vi "SDR.vi"(0 "instrument handle":refnum<k15>="PXI1Slot2 (33)", 1 "Rm (ohm)":dbl=26118.0, 2 "MLC SLV (V)":dbl=2.0, 3 "Step Size":cluster{"WLV":dbl, "BLV":dbl, "SLV":dbl}={"WLV"=0.06, "BLV"=0.4, "SLV"=0.15000000000000002} {"SLV" format="%#_13g"; "BLV" format="%#_13g"; "WLV" format="%#_13g"}, 4 "RM (ohm)":dbl=39476.0, 5 "error in (no error)":errorcluster, 6 "Max fine attempts":i32=20, 8 "RMM (ohm)":dbl=10000000000.0, 9 "Rmm (ohm)":dbl=15300.0, 10 "MLC BLV (V)":dbl=2.0, 11 "MLC WLV (V)":dbl=2.26) -> (7 "BL voltage (V)":dbl=2.8, 12 "SL voltage (V)":dbl=2.15, 13 "WL voltage (V)":dbl=2.26, 14 "instrument handle out":refnum<k15>="PXI1Slot2 (33)", 15 "final resistance (ohm)":dbl=31406.349555562472 format="%#_6p", 17 "target hit?":bool=TRUE, 18 "final current (A)":dbl=6.368139017435645e-06, 19 "error out":errorcluster)   [LabVIEW 2018]
uses:
  Globals.vi
panel:
  out "attempt number":i32=1
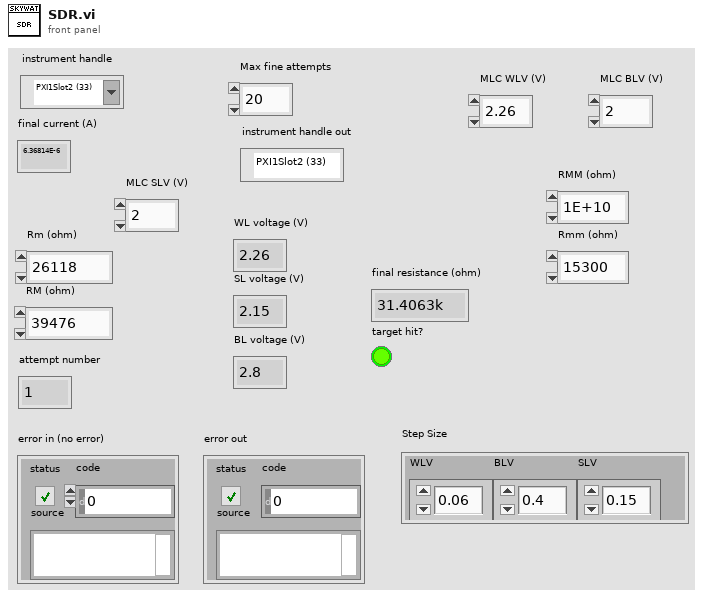
[diagram p1: front panel]
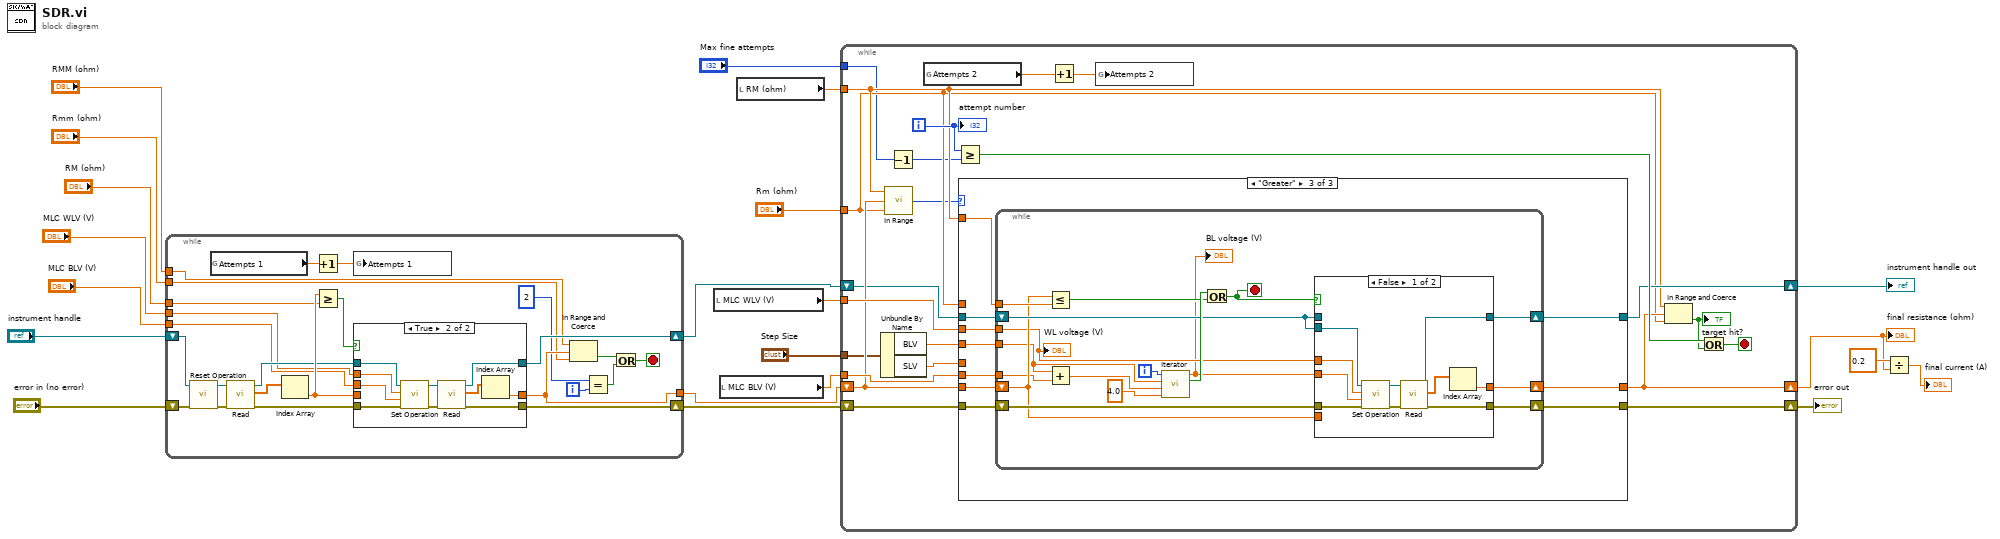
[diagram p0: block diagram]
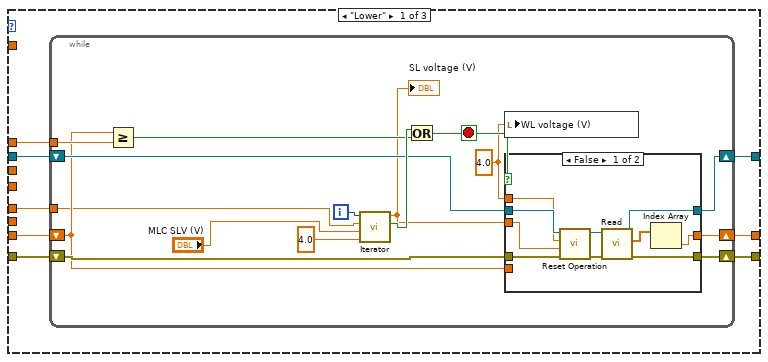
[diagram p3: hidden frame]
diagram:
  n1 = while {
    tunnel: [w36] -> w13
    tunnel: "RM (ohm)" -> [w33]
    shift-right: [w34] -> w11
    shift-left: "error in (no error)" -> [w38]
    shift-right: [w35] -> w12
    shift-left: "instrument handle" -> [w37]
    tunnel: "MLC WLV (V)" -> [w28]
    tunnel: "MLC BLV (V)" -> [w27]
    tunnel: "RMM (ohm)" -> [w26]
    tunnel: "Rmm (ohm)" -> [w25]
    i -> [w30]
    stop <- w32 stop-if-true
    n2 = call "Reset Operation.vi"("error in (no error)"=w38, "instrument handle"=w37) -> ("error out"=w41:errorcluster, "instrument handle out"=w39:refnum<k15>)  [unwired: 8 in]
    n3 = global read "Globals.vi" "Attempts 1"() -> (w23:dbl)
    n4 = call "Read.vi"("error in (no error)"=w41, "instrument handle"=w39) -> ("error out"=w42:errorcluster, "resistances (ohm)"=w40:dbl[], "instrument handle out"=w43:refnum<k15>)  [unwired: 6 in, 1 out]
    n5 = Index Array(array=w40) -> (element=w44:dbl)  [unwired: 1 in]
    n6 = Increment(x=w23) -> (x+1=w22:dbl)
    n7 = Greater Or Equal?(x=w44, y=w33) -> (x >= y?=w45:bool)
    n8 = global write "Globals.vi" "Attempts 1"(w22) -> ()
    n9 = case shown="True" w45 {
      tunnel: w42 -> [w48 w52]
      tunnel: [w48 w54] -> w34
      tunnel: w44 -> [w47 _]
      tunnel: [w47 w55] -> w36
      tunnel: w43 -> [w46 w58]
      tunnel: [w46 w56] -> w35
      tunnel: w28 -> [_ w50]
      tunnel: w27 -> [_ w49]
      frame False {
      }
      frame True {
        n10 = call "Set Operation.vi"("error in (no error)"=w52, "BLV"=w49, "WLV"=w50, "instrument handle"=w58) -> ("error out"=w53:errorcluster, "instrument handle out"=w57:refnum<k15>)  [unwired: 6 in]
        n11 = call "Read.vi"("error in (no error)"=w53, "instrument handle"=w57) -> ("error out"=w54:errorcluster, "resistances (ohm)"=w51:dbl[], "instrument handle out"=w56:refnum<k15>)  [unwired: 6 in, 1 out]
        n12 = Index Array(array=w51) -> (element=w55:dbl)  [unwired: 1 in]
      }
    }
    n13 = In Range and Coerce(upper limit=w26, x=w36, lower limit=w25) -> (In Range?=w24:bool)  [unwired: 1 out]
    n14 = Equal?(x=2, y=w30) -> (x = y?=w31:bool)
    n15 = Or(x=w24, y=w31) -> (x .or. y?=w32:bool)
  }
  n16 = local read "MLC WLV (V)"() -> (w7:dbl)
  n17 = local read "MLC BLV (V)"() -> (w6:dbl)
  n18 = local read "RM (ohm)"() -> (w9:dbl)
  n19 = while {
    shift-right: [w75] -> w16
    shift-left: w12 -> [w69]
    shift-right: [w74] -> w21
    shift-left: w11 -> [w68]
    tunnel: "Max fine attempts" -> [w60]
    tunnel: w9 -> [w71]
    tunnel: w7 -> [w73]
    tunnel: w6 -> [w72]
    tunnel: "Rm (ohm)" -> [w67]
    tunnel: "Step Size" -> [w63]
    shift-right: [w76] -> w18
    shift-left: w13 -> [w70]
    i -> [w79]
    stop <- w80 stop-if-true
    n20 = Unbundle By Name(w63) -> ("BLV"=w65:dbl, "SLV"=w64:dbl)
    n21 = call "In Range.vi"("Lower resistance (ohm)"=w67, "Resistance (ohm)"=w70, "Upper resistance (ohm)"=w71) -> ("range"=w66:enum16{"Lower", "In Range", "Greater"})
    n22 = Decrement(x=w60) -> (x-1=w59:i32)
    n23 = global read "Globals.vi" "Attempts 2"() -> (w61:dbl)
    n24 = Greater Or Equal?(x=w79, y=w59) -> (x >= y?=w78:bool)
    n25 = case shown="\"Greater\"" w66 {
      tunnel: w65 -> [_ _ w130]
      tunnel: w68 -> [w82 w119 w129]
      tunnel: [w86 w119 w128] -> w74
      tunnel: [w87 w120 w127] -> w75
      tunnel: [w81 w118 w123] -> w76
      tunnel: w71 -> [_ _ w126]
      tunnel: w69 -> [w84 w120 w125]
      tunnel: w70 -> [w85 w118 w124]
      tunnel: w67 -> [w88 _ _]
      tunnel: w73 -> [_ _ w122]
      tunnel: w72 -> [_ _ w121]
      tunnel: w64 -> [w83 _ _]
      frame "Lower" {
        n26 = while {
          shift-right: [w99] -> w87
          shift-left: w84 -> [w97]
          shift-right: [w100] -> w86
          shift-left: w82 -> [w98]
          tunnel: w88 -> [w93]
          shift-right: [w91] -> w81
          shift-left: w85 -> [w92]
          tunnel: w83 -> [w90]
          i -> [w104]
          stop <- w96 stop-if-true
          w94 = 4.0 ("level (V)")
          n27 = Greater Or Equal?(x=w92, y=w93) -> (x >= y?=w101:bool)
          n28 = call "Iterator.vi"("Final Value"=4.0 ("y"), "Initial Value"="MLC SLV (V)", "Step"=w90, "i"=w104) -> ("End Loop"=w102:bool, "Current Value"=w95:dbl)  [unwired: 6 in]
          "SL voltage (V)" <- w95
          n29 = Or(x=w102, y=w101) -> (x .or. y?=w96:bool)
          n30 = local write "WL voltage (V)"(w94) -> ()
          n31 = case shown="False" w96 {
            tunnel: w95 -> [w105 _]
            tunnel: [w112 w117] -> w100
            tunnel: [w111 w115] -> w99
            tunnel: w94 -> [w106 _]
            tunnel: w98 -> [w110 w117]
            tunnel: w97 -> [w109 w115]
            tunnel: w92 -> [_ w116]
            tunnel: [w107 w116] -> w91
            frame False {
              n32 = call "Reset Operation.vi"("error in (no error)"=w110, "SLV"=w105, "WLV"=w106, "instrument handle"=w109) -> ("error out"=w113:errorcluster, "instrument handle out"=w114:refnum<k15>)  [unwired: 6 in]
              n33 = call "Read.vi"("error in (no error)"=w113, "instrument handle"=w114) -> ("error out"=w112:errorcluster, "resistances (ohm)"=w108:dbl[], "instrument handle out"=w111:refnum<k15>)  [unwired: 6 in, 1 out]
              n34 = Index Array(array=w108) -> (element=w107:dbl)  [unwired: 1 in]
            }
            frame True {
            }
          }
        }
      }
      frame "In Range", Default {
      }
      frame "Greater" {
        n35 = while {
          shift-right: [w141] -> w127
          shift-left: w125 -> [w139]
          shift-right: [w142] -> w128
          shift-left: w129 -> [w140]
          tunnel: w126 -> [w143]
          tunnel: w130 -> [w131]
          shift-right: [w136] -> w123
          shift-left: w124 -> [w137]
          tunnel: w122 -> [w134]
          tunnel: w121 -> [w133]
          i -> [w147]
          stop <- w138 stop-if-true
          n36 = Less Or Equal?(x=w137, y=w143) -> (x <= y?=w144:bool)
          n37 = Add(x=w131, y=w133) -> (x+y=w135:dbl)
          n38 = call "Iterator.vi"("Final Value"=4.0 ("y"), "Initial Value"=w135, "Step"=w131, "i"=w147) -> ("End Loop"=w145:bool, "Current Value"=w132:dbl)  [unwired: 6 in]
          "BL voltage (V)" <- w132
          n39 = Or(x=w145, y=w144) -> (x .or. y?=w138:bool)
          n40 = case shown="False" w138 {
            tunnel: w134 -> [w157 _]
            tunnel: [w154 w160] -> w142
            tunnel: [w153 w159] -> w141
            tunnel: w132 -> [w152 _]
            tunnel: w140 -> [w151 w160]
            tunnel: w139 -> [w150 _]
            tunnel: w139 -> [_ w159]
            tunnel: w137 -> [_ w158]
            tunnel: [w148 w158] -> w136
            frame False {
              n41 = call "Set Operation.vi"("error in (no error)"=w151, "BLV"=w152, "WLV"=w157, "instrument handle"=w150) -> ("error out"=w155:errorcluster, "instrument handle out"=w156:refnum<k15>)  [unwired: 6 in]
              n42 = call "Read.vi"("error in (no error)"=w155, "instrument handle"=w156) -> ("error out"=w154:errorcluster, "resistances (ohm)"=w149:dbl[], "instrument handle out"=w153:refnum<k15>)  [unwired: 6 in, 1 out]
              n43 = Index Array(array=w149) -> (element=w148:dbl)  [unwired: 1 in]
            }
            frame True {
            }
          }
          "WL voltage (V)" <- w134
        }
      }
    }
    n44 = Increment(x=w61) -> (x+1=w62:dbl)
    n45 = global write "Globals.vi" "Attempts 2"(w62) -> ()
    n46 = In Range and Coerce(upper limit=w71, x=w76, lower limit=w67) -> (In Range?=w77:bool)  [unwired: 1 out]
    "target hit?" <- w77
    n47 = Or(x=w78, y=w77) -> (x .or. y?=w80:bool)
    "attempt number" <- w79
  }
  "error out" <- w21
  "instrument handle out" <- w16
  "final resistance (ohm)" <- w18
  n48 = Divide(x=0.2, y=w18) -> (x/y=→"final current (A)":dbl)
